vi "Write.vi"(8 "error in":errorcluster, 9 "Producer Ch":T1(array[cluster])=[{"Error.STS"=0, "OutputEnable.STS"=0, "ControlMode.STS"=0, "Voltage.AV"=0.0, "Current.AV"=0.0, "Power.AV"=0.0, "VoltageNominal.AV"=0.0, "CurrentNominal.AV"=0.0, "PowerNominal.AV"=0.0, "ParameterSet.STS"=0}], 10 "Producer Control":T2, 11 "Cycler Cluster.lvclass":refnum<class "Cycler Cluster.lvclass">) -> (0 "error out":errorcluster, 3 "Cycler Cluster.lvclass out":refnum<class "Cycler Cluster.lvclass">)   [LabVIEW 2023, in "Cycler Cluster.lvclass"]
uses:
  Cycler Cluster.lvclass
  Cycler Cluster.lvclass/Cycler Cluster.ctl
  6bfc6677-cd67-4f2d-afef-839dec9218ce.vi
  74f11eb1-9425-41af-a169-6608e4aa6674.vi
  6bfc6677-cd67-4f2d-afef-839dec9218ce.vi/4bc1c15b-36ab-481f-b8dd-c64075ce723a.vi
  6bfc6677-cd67-4f2d-afef-839dec9218ce.vi/d83cb72b-7713-41fc-a3d1-682de79cf574.vi
  74f11eb1-9425-41af-a169-6608e4aa6674.vi/4bc1c15b-36ab-481f-b8dd-c64075ce723a.vi
  74f11eb1-9425-41af-a169-6608e4aa6674.vi/d83cb72b-7713-41fc-a3d1-682de79cf574.vi
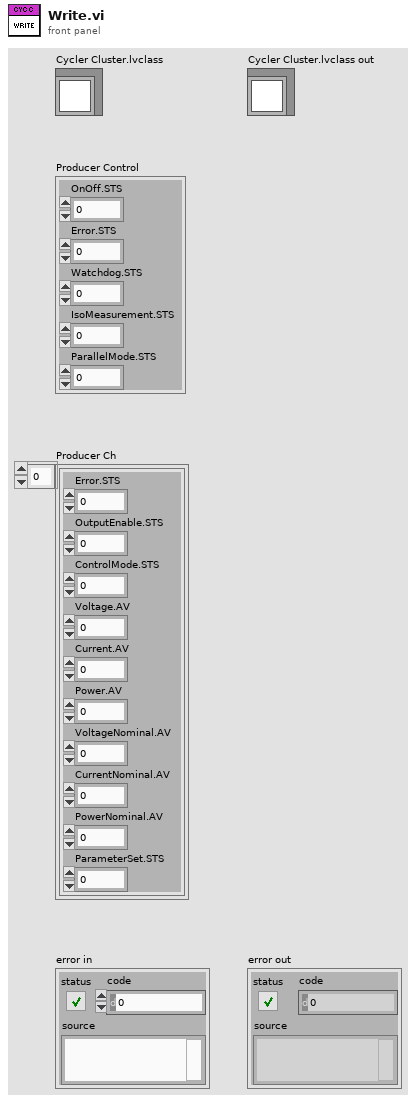
[diagram p1: front panel]
types:
  T1 = cluster{"Error.STS":i32, "OutputEnable.STS":i32, "ControlMode.STS":u16, "Voltage.AV":dbl, "Current.AV":dbl, "Power.AV":dbl, "VoltageNominal.AV":dbl, "CurrentNominal.AV":dbl, "PowerNominal.AV":dbl, "ParameterSet.STS":i32}[]
  T2 = cluster{"OnOff.STS":i32, "Error.STS":i32, "Watchdog.STS":i32, "IsoMeasurement.STS":i32, "ParallelMode.STS":i32}
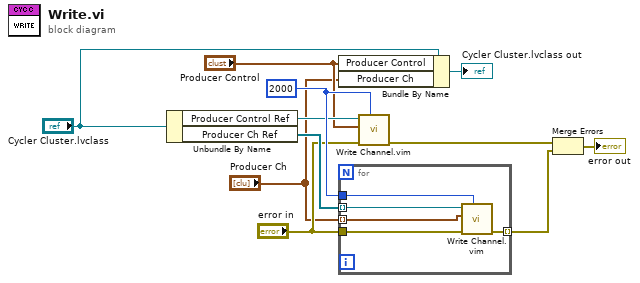
[diagram p0: block diagram]
diagram:
  w8 = 2000 ("Timeout (ms)")
  n1 = Unbundle By Name("Cycler Cluster.lvclass") -> ("Producer Control Ref"=w7:refnum<k21>, "Producer Ch Ref"=w9:refnum<k21>[])
  n2 = Bundle By Name(cluster="Cycler Cluster.lvclass", "Producer Control"="Producer Control", "Producer Ch"="Producer Ch") -> (→"Cycler Cluster.lvclass out":refnum<class "Cycler Cluster.lvclass">)
  n3 = for {
    tunnel: "error in" -> [w16]
    tunnel: [w15] -> w3 mode=indexing
    tunnel: w9 -> [w14] mode=indexing
    tunnel: w8 -> [w13]
    tunnel: "Producer Ch" -> [w12] mode=indexing
    n4 = call "Write Channel.vim"("Timeout (ms)"=w13, "error in"=w16, "Data in"=w12, "ADAS HIL Channel in"=w14) -> ("error out"=w15:errorcluster)  [unwired: 5 in, 2 out]
  }
  n5 = call "Write Channel.vim"("Timeout (ms)"=w8, "error in"="error in", "Data in"="Producer Control", "ADAS HIL Channel in"=w7) -> ("error out"=w4:errorcluster)  [unwired: 5 in, 2 out]
  n6 = Merge Errors(w4, w3) -> (→"error out":errorcluster)
